vi "SetValue.vi"(8 "error in":errorcluster, 10 "Value":u8, 11 "UnsignedByte in":refnum<class "UnsignedByte.lvclass">) -> (0 "error out":errorcluster, 3 "UnsignedByte out":refnum<class "UnsignedByte.lvclass">)   [LabVIEW 2021, in "ProligentXMLGenerator.lvlib" / "UnsignedByte.lvclass"]
uses:
  UnsignedByte.lvclass
  UnsignedByte.lvclass/UnsignedByte.ctl
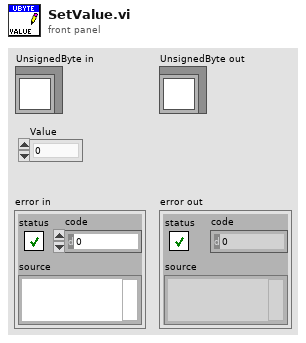
[diagram p1: front panel]
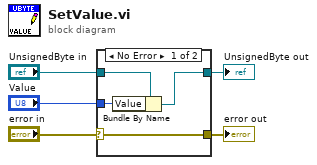
[diagram p0: block diagram]
diagram:
  n1 = case shown="No Error" "error in" {
    selector: "error in" -> [w6 w10]
    tunnel: "UnsignedByte in" -> [w9 w11]
    tunnel: [w8 w11] -> w3
    tunnel: "Value" -> [w7 _]
    tunnel: [w6 w10] -> w2
    frame No Error {
      n2 = Bundle By Name(cluster=w9, "Value"=w7) -> (w8:refnum<class "UnsignedByte.lvclass">)
    }
    frame Error {
    }
  }
  "error out" <- w2
  "UnsignedByte out" <- w3
